vi "run.vi"(8 "error in (no error)":errorcluster, 11 "HGF_DSCMonitor in":refnum<class "HGF_DSCMonitor.lvclass">) -> (0 "error out":errorcluster, 3 "HGF_DSCMonitor out":refnum<class "HGF_DSCMonitor.lvclass">)   [LabVIEW 2012, in "HGF_DSC.lvlib" / "HGF_DSCMonitor.lvclass"]
uses:
  HGF_DSCMonitor.lvclass
  HGF_DSCMonitor.lvclass/HGF_DSCMonitor.ctl
  HGF_BaseClasses/HGF_TriggeredEvent/HGF_TriggeredEvent.lvclass
  HGF_BaseClasses/HGF_NetworkVisitor/HGF_NetworkVisitor.lvclass
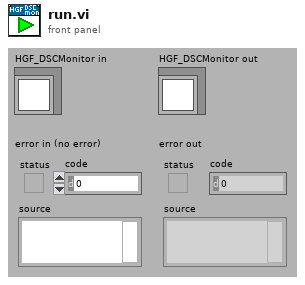
[diagram p1: front panel]
types:
  T1 = cluster{"Shared Variable":refnum<k21>, "registered Visitors":cluster{"HGF_NetworkVisitor":refnum<class "HGF_NetworkVisitor.lvclass">, "HGF_TriggeredEvent":refnum<class "HGF_TriggeredEvent.lvclass">}[]}[]
  T2 = cluster{"Shared Variable":refnum<k21>, "registered Visitors":cluster{"HGF_NetworkVisitor":refnum<class "HGF_NetworkVisitor.lvclass">, "HGF_TriggeredEvent":refnum<class "HGF_TriggeredEvent.lvclass">}[]}
  T3 = cluster{"HGF_NetworkVisitor":refnum<class "HGF_NetworkVisitor.lvclass">, "HGF_TriggeredEvent":refnum<class "HGF_TriggeredEvent.lvclass">}[]
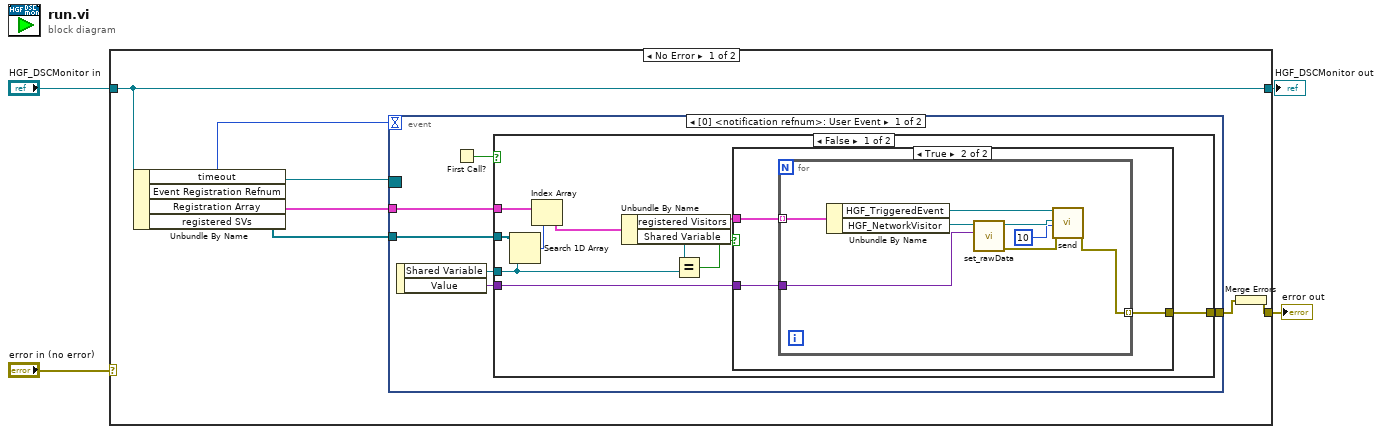
[diagram p0: block diagram]
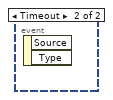
[diagram p4: hidden frame]
diagram:
  n1 = case shown="No Error" "error in (no error)" {
    selector: "error in (no error)" -> [_ w40]
    tunnel: [w5 w40] -> w3
    tunnel: [w9 w39] -> w1
    tunnel: "HGF_DSCMonitor in" -> [w9 w39]
    frame No Error {
      n2 = Unbundle By Name(w9) -> ("timeout"=w7:i32, "Event Registration Refnum"=w10:refnum<event-registration>, "Registration Array"=w8:T1, "registered SVs"=w11:refnum<k21>[])
      n3 = event shown="[0] <notification refnum>: User Event" {
        selector: w10 -> [_ _]
        dyn-events: _ -> [_ _]
        timeout: w7 -> [_ _]
        tunnel: w11 -> [w17 _]
        tunnel: w8 -> [w16 _]
        tunnel: [w13 _] -> w6
        event User Event {
          n4 = event-data() -> ("Shared Variable"=w15:refnum<k21>, "Value"=w12:variant)  [unwired: 1 out]
          n5 = First Call?() -> (First Call?: T/F=w14:bool)
          n6 = case shown="False" w14 {
            tunnel: w17 -> [w27 _]
            tunnel: w16 -> [w26 _]
            tunnel: w15 -> [w19 _]
            tunnel: [w20 _] -> w13
            tunnel: w12 -> [w18 _]
            frame False {
              n7 = Search 1D Array(1D array=w27, element=w19) -> (index of element=w25:i32)  [unwired: 1 out]
              n8 = Index Array(array=w26, index=w25) -> (element=w24:T2)
              n9 = Unbundle By Name(w24) -> ("registered Visitors"=w21:T3, "Shared Variable"=w23:refnum<k21>)
              n10 = Equal?(x=w23, y=w19) -> (x = y?=w22:bool)
              n11 = case shown="True" w22 {
                tunnel: w21 -> [_ w30]
                tunnel: [_ w28] -> w20
                tunnel: w18 -> [_ w29]
                frame False {
                }
                frame True {
                  n12 = for {
                    tunnel: w30 -> [w38] mode=indexing
                    tunnel: w29 -> [w34]
                    tunnel: [w31] -> w28 mode=indexing
                    n13 = Unbundle By Name(w38) -> ("HGF_TriggeredEvent"=w33:refnum<class "HGF_TriggeredEvent.lvclass">, "HGF_NetworkVisitor"=w36:refnum<class "HGF_NetworkVisitor.lvclass">)
                    n14 = call "set_rawData.vi"("rawData"=w34, "HGF_NetworkData"=w36) -> ("error out"=w37:errorcluster, "dup HGF_NetworkData"=w35:refnum<class "HGF_NetworkVisitor.lvclass">)  [unwired: 1 in, 7 out]
                    n15 = call-dynamic "send.vi"("HGF_Event"=w33, "Object"=w35, "timeout in ms (-1)"=10, "error in (no error)"=w37) -> ("error out"=w31:errorcluster)  [unwired: 13 in, 2 out]
                  }
                }
              }
            }
            frame True {
            }
          }
        }
        event Timeout {
          n16 = event-data() -> ()  [unwired: 3 out]
        }
      }
      n17 = Merge Errors(w6) -> (w5:errorcluster)
    }
    frame Error {
    }
  }
  "error out" <- w3
  "HGF_DSCMonitor out" <- w1
